vi "Unit Vector.vi"   [LabVIEW 2020, in "NI_AALBase.lvlib"]
doc: "Finds the <B>norm</B> of the <B>Input Vector</B> and obtains its corresponding <B>Unit Vector</B> by normalizing the original <B>Input Vector</B> with its <B>norm</B>."
uses:
  <vilib>/Analysis/NI_AALBase.lvlib
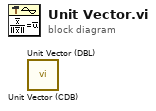
[diagram p0: block diagram]
diagram:
  n1 = call <vilib>:"Unit Vector (CDB).vi"() -> ()  [unwired: 9 in, 3 out]
  n2 = call <vilib>:"Unit Vector (DBL).vi"() -> ()  [unwired: 9 in, 3 out]
